vi "Filter And List Panes.vi"(8 "Error In":errorcluster, 10 "Splitter Refs":refnum<vi>[](array[refnum]), 11 "Control Reference Lists In":T1) -> (0 "Error Out":errorcluster, 3 "Control Reference Lists Out":T1)   [LabVIEW 2021, in "Appearance Actor.lvlib" / "Appearance Actor.lvclass"]
uses:
  Appearance Actor.lvclass
  Typedefs/Control Reference Lists--cluster.ctl
  Typedefs/Control Reference Lists-TitleBar--cluster.ctl
  Typedefs/Control Reference Lists-SideMenu--cluster.ctl
  Typedefs/Control Reference Lists-BodyPane--cluster.ctl
  Typedefs/Control Reference Lists-StatusBar--cluster.ctl
  <vilib>/regexp/Match Regular Expression.xnode
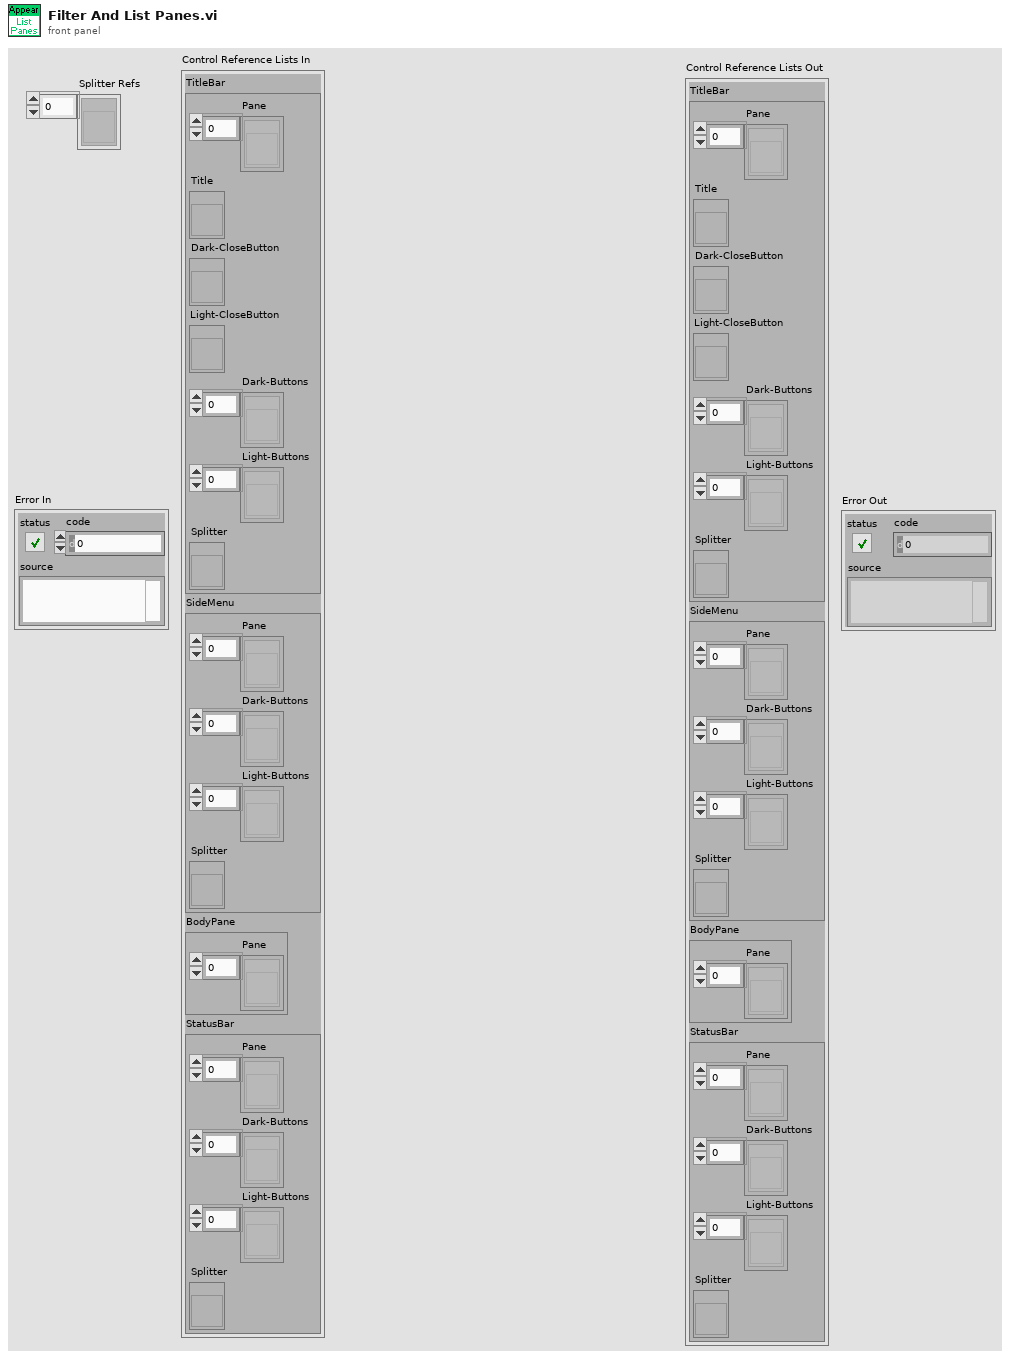
[diagram p1: front panel]
types:
  T1 = typedef "Appearance Actor.lvlib/Appearance Actor.lvclass/Control Reference Lists--cluster.ctl" = cluster{"TitleBar":T2, "SideMenu":T3, "BodyPane":T4, "StatusBar":T5}
  T2 = typedef "Appearance Actor.lvlib/Appearance Actor.lvclass/Control Reference Lists-TitleBar--cluster.ctl" = cluster{"Pane":refnum<vi>[], "Title":refnum<vi>, "Dark-CloseButton":refnum<vi>, "Light-CloseButton":refnum<vi>, "Dark-Buttons":refnum<vi>[], "Light-Buttons":refnum<vi>[], "Splitter":refnum<vi>}
  T3 = typedef "Appearance Actor.lvlib/Appearance Actor.lvclass/Control Reference Lists-SideMenu--cluster.ctl" = cluster{"Pane":refnum<vi>[], "Dark-Buttons":refnum<vi>[], "Light-Buttons":refnum<vi>[], "Splitter":refnum<vi>}
  T4 = typedef "Appearance Actor.lvlib/Appearance Actor.lvclass/Control Reference Lists-BodyPane--cluster.ctl" = cluster{"Pane":refnum<vi>[]}
  T5 = typedef "Appearance Actor.lvlib/Appearance Actor.lvclass/Control Reference Lists-StatusBar--cluster.ctl" = cluster{"Pane":refnum<vi>[], "Dark-Buttons":refnum<vi>[], "Light-Buttons":refnum<vi>[], "Splitter":refnum<vi>}
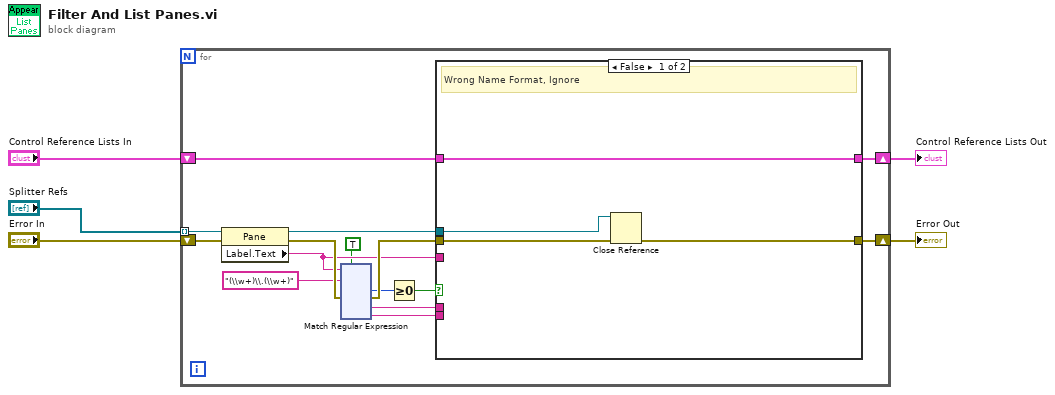
[diagram p0: block diagram]
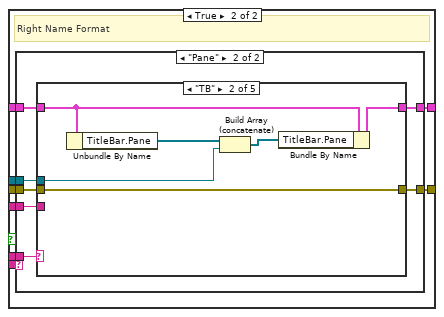
[diagram p2: hidden frame]
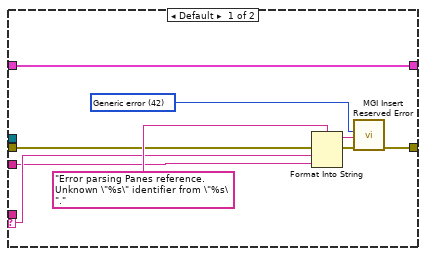
[diagram p3: hidden frame]
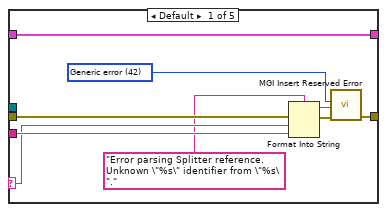
[diagram p4: hidden frame]
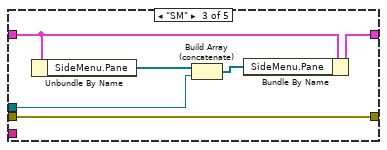
[diagram p5: hidden frame]
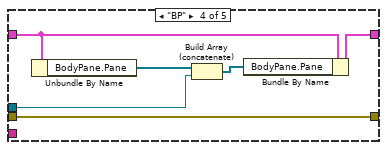
[diagram p6: hidden frame]
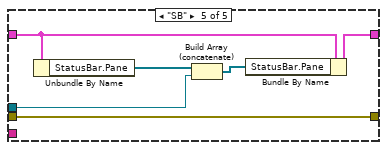
[diagram p7: hidden frame]
diagram:
  n1 = for {
    tunnel: "Splitter Refs" -> [w20] mode=indexing
    shift-right: [w13] -> w1
    shift-left: "Error In" -> [w19]
    shift-right: [w15] -> w2
    shift-left: "Control Reference Lists In" -> [w17]
    n2 = property class="Pane"(reference=w20, error in=w19) -> (reference out=w8:refnum<vi>, error out=w18:errorcluster, "Label.Text"=w11:string)
    n3 = xnode "Match Regular Expression"("input string"=w11, "regular expression"="(\\w+)\\.(\\w+)", "error in"=w18, "ignore case? (F)"=TRUE) -> ("offset past match"=w7:i32, "error out"=w14:errorcluster, "submatch 1"=w16:string, "submatch 2"=w9:string)  [unwired: 2 in, 3 out]
    n4 = Greater Or Equal To 0?(x=w7) -> (x >= 0?=w6:bool)
    n5 = case shown="False" w6 {
      tunnel: w17 -> [w24 w32]
      tunnel: w16 -> [_ w31]
      tunnel: [w24 w30] -> w15
      tunnel: w14 -> [w23 w29]
      tunnel: [w21 w28] -> w13
      tunnel: w11 -> [_ w27]
      tunnel: w9 -> [_ w26]
      tunnel: w8 -> [w22 w25]
      frame False {
        # "Wrong Name Format, Ignore"
        n6 = Close Reference(reference=w22, error in (no error)=w23) -> (error out=w21:errorcluster)
      }
      frame True {
        # "Right Name Format"
        n7 = case shown="\"Pane\"" w26 {
          selector: w26 -> [w34 _]
          tunnel: w32 -> [w41 w48]
          tunnel: w31 -> [_ w47]
          tunnel: [w41 w46] -> w30
          tunnel: w29 -> [w36 w45]
          tunnel: [w35 w44] -> w28
          tunnel: w27 -> [w33 w43]
          tunnel: w25 -> [_ w42]
          frame Default {
            w38 = 42 items=["No error", "Argument error", "Memory is full", "Out of zone", "End of file", "File already open", "Generic file I/O error", "File not found", "File permission error", "Disk is full", "Duplicate path", "Too many files open", "System feature not enabled", "Resource file not found", "Cannot add resource", "Resource not found", "Image not found", "Image memory error", "Pen does not exist", "Config type invalid", "Config token not found", "Config parse error", "Config memory error", "Bad external code format", "Bad external code offset", "External code not present", "Null window", "Destroy window error", "Null menu", "Print aborted", "Bad print record", "Print driver error", "Windows error during printing", "Memory error during printing", "Print dialog error", "Generic print error", "Invalid device refnum", "Device not found", "Device parameter error", "Device unit error", "Cannot open device", "Device call aborted", "Generic error", "Cancelled by user", "Object ID too low", "Object ID too high", "Object not in heap", "Unknown heap", "Unknown object (invalid DefProc)", "Unknown object (DefProc not in table)", "Message out of range", "Invalid (null) method", "Unknown message", "Manager call not supported", "Bad address", "Network operation in progress", "Network operation timed out", "Connection is busy", "Network attribute not supported", "Network error", "Address in use", "System out of memory", "Connection aborted", "Connection refused", "Not connected", "Already connected", "Connection closed", "Initialization error (interapplication manager)", "Bad occurrence", "Wait on unbound occurrence handler", "Occurrence queue overflow", "Datalog type conflict", "Unused", "Unrecognized type (interapplication manager)", "Memory corrupt", "Failed to make temporary DLL", "Old CIN version", "Drag socket not found", "Failed to load drop-object", "Failed to register OLE object", "Failed to release OLE object", "Format specifier type mismatch", "Unknown format specifier", "Too few format specifiers", "Too many format specifiers", "Scan failed", "Newer CIN version", "OLE Convert", "Runtime menu error", "Password tampered", "Unknown error code"] ("Reserved Error Code (Generic error)")
            # "SubSplitter or other"
            n8 = Format Into String(format string="Error parsing Panes reference. Unknown \"%s\" identifier from \"%s\".", error in=w36, w34, w33) -> (resulting string=w40:string, error out=w39:errorcluster)  [unwired: 1 in]
            n9 = call <userlib>:"MGI Insert Reserved Error.vi"("Error In"=w39, "Error Description"=w40, "Reserved Error Code (Generic error)"=w38) -> ("Error Out"=w35:errorcluster)  [unwired: 8 in]
          }
          frame "Pane" {
            # "Splitter"
            n10 = case shown="\"TB\"" w47 {
              selector: w47 -> [w50 _ _ _ _]
              tunnel: w48 -> [w57 w61 w67 w73 w79]
              tunnel: [w57 w63 w69 w75 w81] -> w46
              tunnel: w45 -> [w53 w62 w68 w74 w80]
              tunnel: [w52 w62 w68 w74 w80] -> w44
              tunnel: w43 -> [w51 _ _ _ _]
              tunnel: w42 -> [_ w58 w64 w70 w76]
              frame Default {
                w54 = 42 items=["No error", "Argument error", "Memory is full", "Out of zone", "End of file", "File already open", "Generic file I/O error", "File not found", "File permission error", "Disk is full", "Duplicate path", "Too many files open", "System feature not enabled", "Resource file not found", "Cannot add resource", "Resource not found", "Image not found", "Image memory error", "Pen does not exist", "Config type invalid", "Config token not found", "Config parse error", "Config memory error", "Bad external code format", "Bad external code offset", "External code not present", "Null window", "Destroy window error", "Null menu", "Print aborted", "Bad print record", "Print driver error", "Windows error during printing", "Memory error during printing", "Print dialog error", "Generic print error", "Invalid device refnum", "Device not found", "Device parameter error", "Device unit error", "Cannot open device", "Device call aborted", "Generic error", "Cancelled by user", "Object ID too low", "Object ID too high", "Object not in heap", "Unknown heap", "Unknown object (invalid DefProc)", "Unknown object (DefProc not in table)", "Message out of range", "Invalid (null) method", "Unknown message", "Manager call not supported", "Bad address", "Network operation in progress", "Network operation timed out", "Connection is busy", "Network attribute not supported", "Network error", "Address in use", "System out of memory", "Connection aborted", "Connection refused", "Not connected", "Already connected", "Connection closed", "Initialization error (interapplication manager)", "Bad occurrence", "Wait on unbound occurrence handler", "Occurrence queue overflow", "Datalog type conflict", "Unused", "Unrecognized type (interapplication manager)", "Memory corrupt", "Failed to make temporary DLL", "Old CIN version", "Drag socket not found", "Failed to load drop-object", "Failed to register OLE object", "Failed to release OLE object", "Format specifier type mismatch", "Unknown format specifier", "Too few format specifiers", "Too many format specifiers", "Scan failed", "Newer CIN version", "OLE Convert", "Runtime menu error", "Password tampered", "Unknown error code"] ("Reserved Error Code (Generic error)")
                n11 = Format Into String(format string="Error parsing Splitter reference. Unknown \"%s\" identifier from \"%s\".", error in=w53, w50, w51) -> (resulting string=w56:string, error out=w55:errorcluster)  [unwired: 1 in]
                n12 = call <userlib>:"MGI Insert Reserved Error.vi"("Error In"=w55, "Error Description"=w56, "Reserved Error Code (Generic error)"=w54) -> ("Error Out"=w52:errorcluster)  [unwired: 8 in]
              }
              frame "TB" {
                n13 = Unbundle By Name(w61) -> ("TitleBar.Pane"=w60:refnum<vi>[])
                n14 = Build Array (concatenate)(w60, w58) -> (w59:refnum<vi>[])
                n15 = Bundle By Name(cluster=w61, "TitleBar.Pane"=w59) -> (w63:T1)
              }
              frame "SM" {
                n16 = Unbundle By Name(w67) -> ("SideMenu.Pane"=w66:refnum<vi>[])
                n17 = Build Array (concatenate)(w66, w64) -> (w65:refnum<vi>[])
                n18 = Bundle By Name(cluster=w67, "SideMenu.Pane"=w65) -> (w69:T1)
              }
              frame "BP" {
                n19 = Unbundle By Name(w73) -> ("BodyPane.Pane"=w72:refnum<vi>[])
                n20 = Build Array (concatenate)(w72, w70) -> (w71:refnum<vi>[])
                n21 = Bundle By Name(cluster=w73, "BodyPane.Pane"=w71) -> (w75:T1)
              }
              frame "SB" {
                n22 = Unbundle By Name(w79) -> ("StatusBar.Pane"=w78:refnum<vi>[])
                n23 = Build Array (concatenate)(w78, w76) -> (w77:refnum<vi>[])
                n24 = Bundle By Name(cluster=w79, "StatusBar.Pane"=w77) -> (w81:T1)
              }
            }
          }
        }
      }
    }
  }
  "Error Out" <- w1
  "Control Reference Lists Out" <- w2
